vi "General-Update_t0.vi"(2 "#samples":u32, 3 "t0 IN":timestamp, 4 "dt":dbl) -> (0 "tf new":timestamp, 1 "t0 OUT":timestamp)   [LabVIEW 2010]
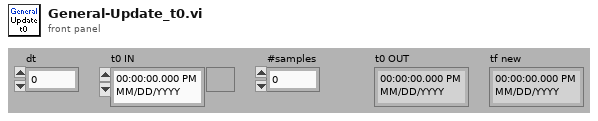
[diagram p1: front panel]
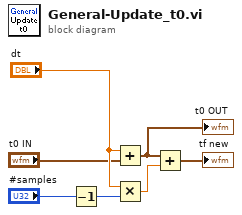
[diagram p0: block diagram]
diagram:
  n1 = Decrement(x="#samples") -> (x-1=w1:u32)
  n2 = Add(x="dt", y="t0 IN") -> (x+y=w5:timestamp)
  "t0 OUT" <- w5
  n3 = Multiply(x="dt", y=w1) -> (x*y=w6:dbl)
  n4 = Add(x=w5, y=w6) -> (x+y=→"tf new":timestamp)
